vi "loadTableModel.vi"(8 "error in (no error)":errorcluster, 11 "Game in":refnum<class "Game.lvclass">) -> (0 "error out":errorcluster, 2 "array":dbl[][](array[numeric]), 3 "Game out":refnum<class "Game.lvclass">)   [LabVIEW 2021, in "Game.lvclass"]
uses:
  Game.lvclass
  Utilities_class/Utilities.lvclass
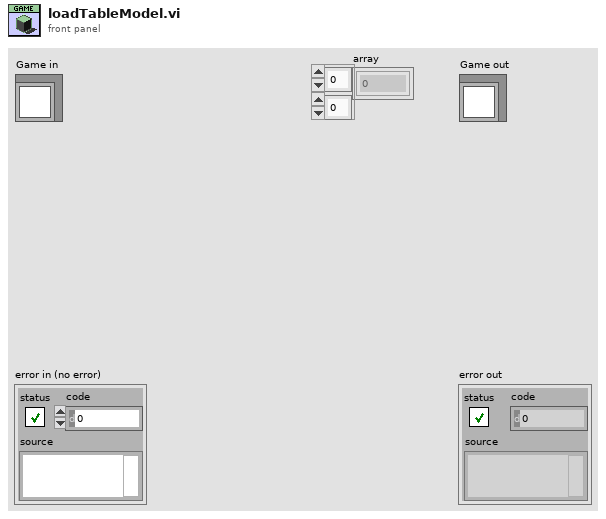
[diagram p1: front panel]
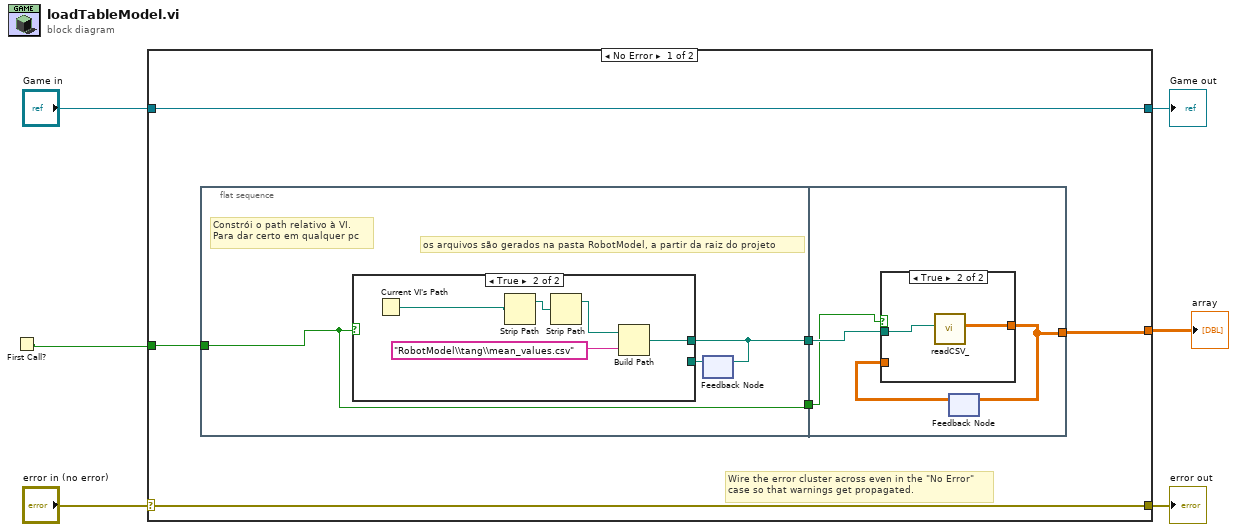
[diagram p0: block diagram]
diagram:
  n1 = First Call?() -> (First Call?: T/F=w1:bool)
  n2 = case shown="No Error" "error in (no error)" {
    selector: "error in (no error)" -> [w11 w30]
    tunnel: [w11 w30] -> w5
    tunnel: [w12 w29] -> w3
    tunnel: "Game in" -> [w12 w29]
    tunnel: [w8 _] -> w2
    tunnel: w1 -> [w7 _]
    frame No Error {
      # "Wire the error cluster across even in the \"No Error\"\ncase so that warnings get propagated."
      n3 = flat-sequence {
        tunnel: [w14] -> w10
        tunnel: [w13] -> w9
        tunnel: w7 -> [w13]
        tunnel: w10 -> [w25]
        tunnel: w9 -> [w24]
        tunnel: [w22] -> w8
        frame #0 {
          # "os arquivos são gerados na pasta RobotModel, a partir da raiz do projeto"
          # "Constrói o path relativo à VI.\nPara dar certo em qualquer pc"
          n4 = feedback #1() -> (w15:path)  [unwired: 1 in]
          n5 = case shown="True" w13 {
            tunnel: [w16 w19] -> w14
            tunnel: w15 -> [w16 _]
            frame False {
              # "só precisa calcular o path na 1° iteração"
            }
            frame True {
              n6 = Current VI's Path() -> (path=w17:path)
              n7 = Strip Path(path=w17) -> (stripped path=w20:path)  [unwired: 1 out]
              n8 = Strip Path(path=w20) -> (stripped path=w18:path)  [unwired: 1 out]
              n9 = Build Path(base path=w18, name or relative path="RobotModel\\tang\\mean_values.csv") -> (appended path=w19:path)
            }
          }
          n10 = feedback-in #1(w14) -> ()
        }
        frame #1 {
          n11 = feedback #2() -> (w23:dbl[][])  [unwired: 1 in]
          n12 = case shown="True" w24 {
            tunnel: w25 -> [_ w28]
            tunnel: [w26 w27] -> w22
            tunnel: w23 -> [w26 _]
            frame False {
            }
            frame True {
              n13 = call "readCSV_.vi"("file path (use dialog)"=w28) -> ("array"=w27:dbl[][])  [unwired: 8 in, 2 out]
            }
          }
          n14 = feedback-in #2(w22) -> ()
        }
      }
    }
    frame Error {
    }
  }
  "error out" <- w5
  "Game out" <- w3
  "array" <- w2
